vi "(SubVI)_PolyEval.vi"(9 "Poly Coefficients":dbl[](array[numeric]), 10 "No Of Coeffs":i32, 11 "Optical Power (mW)":dbl) -> (3 "Voltage (V)":dbl)   [LabVIEW 2019]
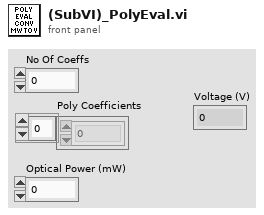
[diagram p1: front panel]
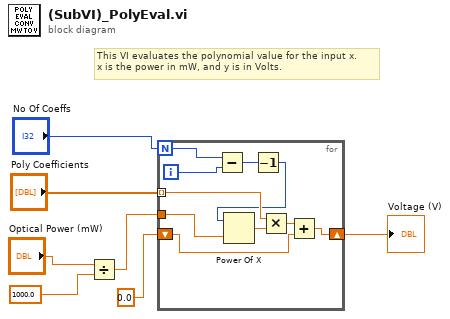
[diagram p0: block diagram]
diagram:
  # "This VI evaluates the polynomial value for the input x.\nx is the power in mW, and y is in Volts."
  n1 = Divide(x="Optical Power (mW)", y=1000.0) -> (x/y=w3:dbl)
  n2 = for {
    N: "No Of Coeffs" -> [w11]
    tunnel: "Poly Coefficients" -> [w15] mode=indexing
    shift-right: [w12] -> w4
    shift-left: 0.0 -> [w13]
    tunnel: w3 -> [w17]
    i -> [w10]
    n3 = Subtract(x=w11, y=w10) -> (x-y=w9:i32)
    n4 = Decrement(x=w9) -> (x-1=w8:i32)
    n5 = Power Of X(1:w17, 2:w8) -> (0:w16:dbl)
    n6 = Multiply(x=w15, y=w16) -> (x*y=w14:dbl)
    n7 = Add(x=w14, y=w13) -> (x+y=w12:dbl)
  }
  "Voltage (V)" <- w4
